vi "Set_VI_Page_Header_Options.vi"(2 "error in":errorcluster, 3 "page header options":T1={"page headers (unchanged)"=0, "page header content options"={"Include VI Name"=TRUE, "Include VI Path"=TRUE, "Include Last Modification Date"=TRUE, "Include Date Printed"=TRUE, "Include Page Number"=TRUE, "Include VI Icon"=TRUE}} {"page headers (unchanged)" items=["Unchanged", "Include page headers", "Do not include page headers"]}, 4 "VI Refnum":refnum<vi>) -> (0 "error out":errorcluster, 1 "VI Refnum out":refnum<vi>)   [LabVIEW 2017, in "NI_ReportGenerationCore.lvlib"]
uses:
  <vilib>/Utility/NIReport.llb/NI_ReportGenerationCore.lvlib
  <vilib>/printing/EasyPrintingControls.llb/page_header_options.ctl
  <vilib>/printing/EasyPrintingControls.llb/page_headers.ctl
  <vilib>/printing/EasyPrintingControls.llb/page_header_content_options.ctl
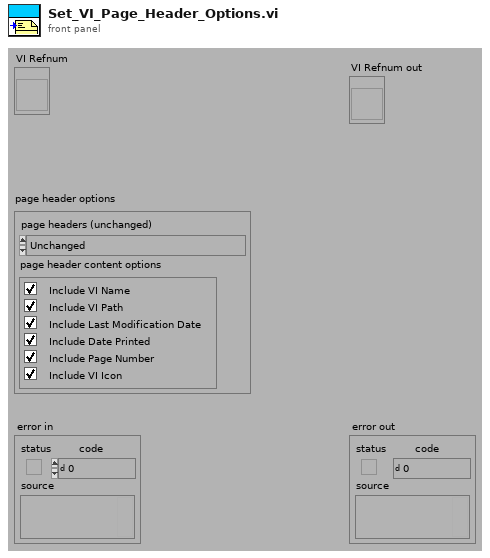
[diagram p1: front panel]
types:
  T1 = typedef "NI_ReportGenerationCore.lvlib/page_header_options.ctl" = cluster{"page headers (unchanged)":T2, "page header content options":T3}
  T2 = typedef "NI_ReportGenerationCore.lvlib/page_headers.ctl" = u16
  T3 = typedef "NI_ReportGenerationCore.lvlib/page_header_content_options.ctl" = cluster{"Include VI Name":bool, "Include VI Path":bool, "Include Last Modification Date":bool, "Include Date Printed":bool, "Include Page Number":bool, "Include VI Icon":bool}
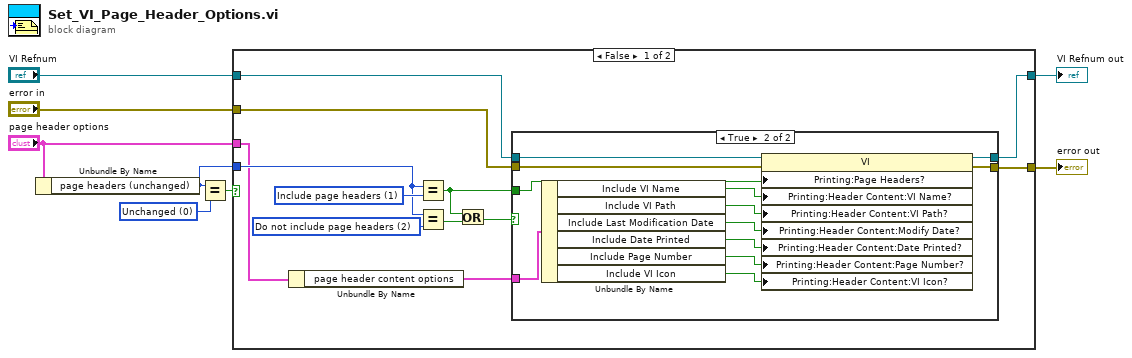
[diagram p0: block diagram]
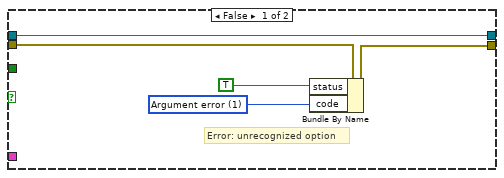
[diagram p2: hidden frame]
diagram:
  w2 = T2 0 items=["Unchanged", "Include page headers", "Do not include page headers"] ("page headers (unchanged)")
  n1 = Unbundle By Name("page header options") -> ("page headers (unchanged)"=w3:T2)
  n2 = Equal?(x=w3, y=w2) -> (x = y?=w4:bool)
  n3 = case shown="False" w4 {
    tunnel: "VI Refnum" -> [w16 w39]
    tunnel: "error in" -> [w18 w38]
    tunnel: [w17 w38] -> w8
    tunnel: [w15 w39] -> w5
    tunnel: "page header options" -> [w11 _]
    tunnel: w3 -> [w12 _]
    frame False {
      w14 = T2 2 items=["Unchanged", "Include page headers", "Do not include page headers"] ("page headers (unchanged)")
      w13 = T2 1 items=["Unchanged", "Include page headers", "Do not include page headers"] ("page headers (unchanged)")
      n4 = Unbundle By Name(w11) -> ("page header content options"=w10:T3)
      n5 = Equal?(x=w12, y=w13) -> (x = y?=w9:bool)
      n6 = Equal?(x=w12, y=w14) -> (x = y?=w20:bool)
      n7 = Or(x=w9, y=w20) -> (x .or. y?=w19:bool)
      n8 = case shown="True" w19 {
        tunnel: w18 -> [w23 w36]
        tunnel: [w21 w34] -> w17
        tunnel: w16 -> [w22 w37]
        tunnel: [w22 w35] -> w15
        tunnel: w10 -> [_ w32]
        tunnel: w9 -> [_ w33]
        frame False {
          w24 = 1 items=["No error", "Argument error", "Memory is full", "Out of zone", "End of file", "File already open", "Generic file I/O error", "File not found", "File permission error", "Disk is full", "Duplicate path", "Too many files open", "System feature not enabled", "Resource file not found", "Cannot add resource", "Resource not found", "Image not found", "Image memory error", "Pen does not exist", "Config type invalid", "Config token not found", "Config parse error", "Config memory error", "Bad external code format", "Bad external code offset", "External code not present", "Null window", "Destroy window error", "Null menu", "Print aborted", "Bad print record", "Print driver error", "Windows error during printing", "Memory error during printing", "Print dialog error", "Generic print error", "Invalid device refnum", "Device not found", "Device parameter error", "Device unit error", "Cannot open device", "Device call aborted", "Generic error", "Cancelled by user", "Object ID too low", "Object ID too high", "Object not in heap", "Unknown heap", "Unknown object (invalid DefProc)", "Unknown object (DefProc not in table)", "Message out of range", "Invalid (null) method", "Unknown message", "Manager call not supported", "Bad address", "Network operation in progress", "Network operation timed out", "Connection is busy", "Network attribute not supported", "Network error", "Address in use", "System out of memory", "Connection aborted", "Connection refused", "Not connected", "Already connected", "Connection closed", "Initialization error (interapplication manager)", "Bad occurrence", "Wait on unbound occurrence handler", "Occurrence queue overflow", "Datalog type conflict", "Unused", "Unrecognized type (interapplication manager)", "Memory corrupt", "Failed to make temporary DLL", "Old CIN version", "Drag socket not found", "Failed to load drop-object", "Failed to register OLE object", "Failed to release OLE object", "Format specifier type mismatch", "Unknown format specifier", "Too few format specifiers", "Too many format specifiers", "Scan failed", "Newer CIN version", "Error converting to variant", "Runtime menu error", "Password tampered", "Variant attribute not found", "Incompatible variant data type", "Event data is not available", "Event Store is not present", "Occurrence is not found", "Event Queue is not created", "Event info is not available", "Refnum passed is NULL", "Error retrieving Class GUID", "Error retrieving CoClass GUID", "Error retrieving TypeLib GUID.", "Bad built application magic bytes.", "Specific driver is different from the specific driver associated with the Logical Name.", "There is no session opened to the class driver.", "Max Error", "MAX - Error with config objects", "MAX - Error loading configuration", "MAX - Group not supported"]
          # "Error: unrecognized option"
          n9 = Bundle By Name(cluster=w23, "status"=TRUE, "code"=w24) -> (w21:errorcluster)
        }
        frame True {
          n10 = Unbundle By Name(w32) -> ("Include VI Name"=w31:bool, "Include VI Path"=w30:bool, "Include Last Modification Date"=w29:bool, "Include Date Printed"=w28:bool, "Include Page Number"=w27:bool, "Include VI Icon"=w26:bool)
          n11 = property class="VI"(reference=w37, error in=w36, "Printing:Page Headers?"=w33, "Printing:Header Content:VI Name?"=w31, "Printing:Header Content:VI Path?"=w30, "Printing:Header Content:Modify Date?"=w29, "Printing:Header Content:Date Printed?"=w28, "Printing:Header Content:Page Number?"=w27, "Printing:Header Content:VI Icon?"=w26) -> (reference out=w35:refnum<vi>, error out=w34:errorcluster)
        }
      }
    }
    frame True {
      # "Do not change this setting"
    }
  }
  "VI Refnum out" <- w5
  "error out" <- w8
